vi "Query Generator Trigger Source Catalog.vi"(8 "error in (no error)":errorcluster, 10 "Instance (1)":i32=1, 11 "VISA resource name":refnum<visa-resource-name>) -> (0 "error out":errorcluster, 2 "Catalog":string, 3 "VISA resource name out":refnum<visa-resource-name>)   [LabVIEW 2015, in "Rohde&Schwarz CMXP GPRF.lvlib"]
doc: "Lists all trigger source values that can be set using TRIGger:GPRF:GEN<i>[:ARB]:SOURce.\n\nAttribute(s):\nRSCMXPGPRF_ATTR_BASEBAND_TRIGGER_CATALOG_SOURCE\n\nRemote-control command(s):\nTRIGger:GPRF:GEN<i>[:ARB]:CATalog:SOURce?"
uses:
  <instrlib>/Rohde&Schwarz CMXP GPRF/Rohde&Schwarz CMXP GPRF.lvlib
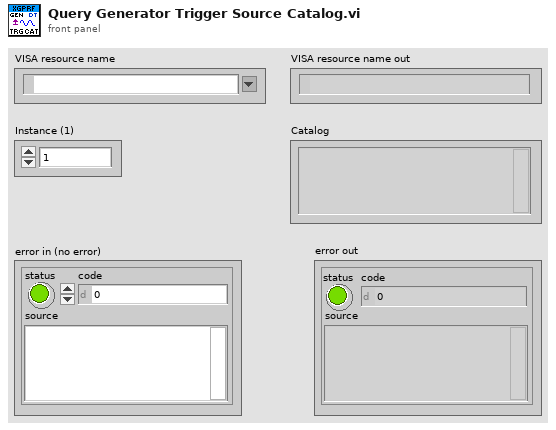
[diagram p1: front panel]
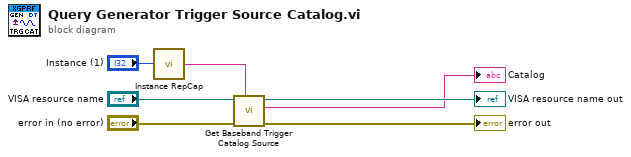
[diagram p0: block diagram]
diagram:
  n1 = call <instrlib>:"Instance RepCap.vi"("instance  in"="Instance (1)") -> ("instance out"=w3:string)
  n2 = call "Get Baseband Trigger Catalog Source"("Repeated Capabilities"=w3, "error in (no error)"="error in (no error)", "instrument handle"="VISA resource name") -> ("error out"=→"error out":errorcluster, "Baseband Trigger Catalog Source"=→"Catalog":string, "instrument handle out"=→"VISA resource name out":refnum<visa-resource-name>)  [unwired: 6 in]
